vi "Build Boolean Filter.vi"(8 "error in (no error)":errorcluster, 10 "Comparision Value":bool, 11 "Boolean Filter in":refnum<class "Boolean Filter.lvclass">) -> (0 "error out":errorcluster, 3 "Boolean Filter out":refnum<class "Boolean Filter.lvclass">)   [LabVIEW 2016, in "Assert API Components.lvlib" / "Boolean Filter.lvclass"]
uses:
  Boolean Filter.lvclass
  Boolean Filter.lvclass/Boolean Filter.ctl
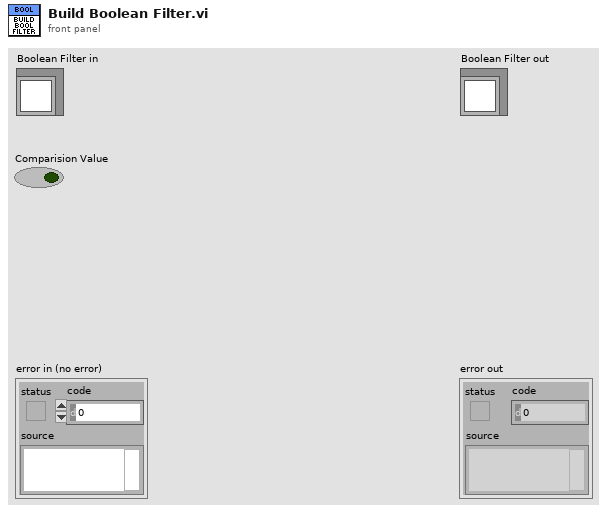
[diagram p1: front panel]
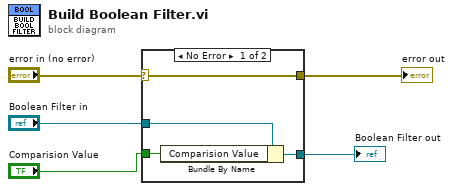
[diagram p0: block diagram]
diagram:
  n1 = case shown="No Error" "error in (no error)" {
    selector: "error in (no error)" -> [w8 w11]
    tunnel: [w8 w11] -> w4
    tunnel: [w7 w10] -> w2
    tunnel: "Boolean Filter in" -> [w9 w10]
    tunnel: "Comparision Value" -> [w6 _]
    frame No Error {
      n2 = Bundle By Name(cluster=w9, "Comparision Value"=w6) -> (w7:refnum<class "Boolean Filter.lvclass">)
    }
    frame Error {
    }
  }
  "error out" <- w4
  "Boolean Filter out" <- w2
